vi "rqcBob ServiceNET Read Data.vi"(8 "error in":errorcluster, 11 "rqcBob ServiceNET in":T1) -> (0 "error out":errorcluster, 1 "data valid":bool, 2 "Data":u32[](array[numeric]), 3 "rqcBob ServiceNET out":T1)   [LabVIEW 2018]
uses:
  Custom Controls/rqcBob ServiceNET control.ctl
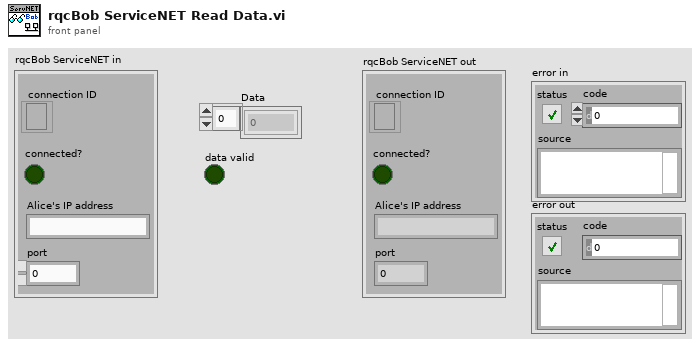
[diagram p1: front panel]
types:
  T1 = typedef "rqcBob ServiceNET control.ctl" = cluster{"connection ID":refnum<k5>, "connected?":bool, "Alice's IP address":string, "port":u16}
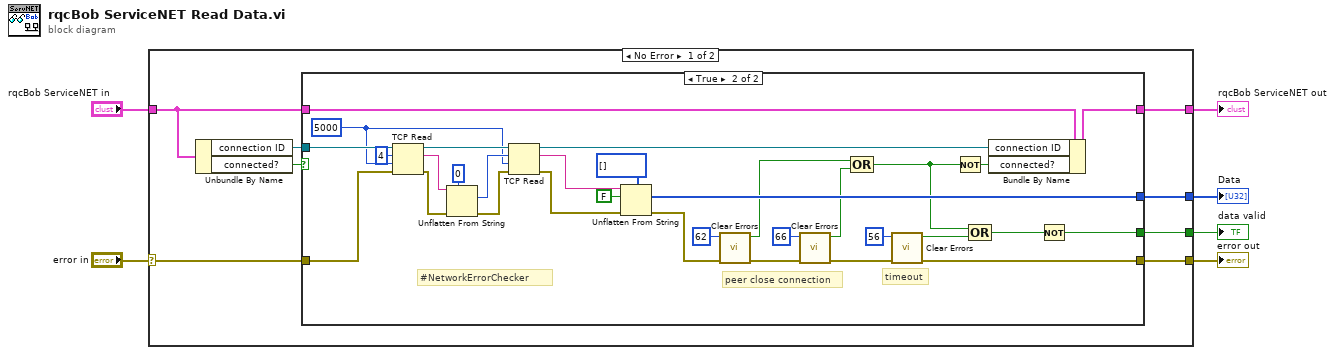
[diagram p0: block diagram]
diagram:
  n1 = case shown="No Error" "error in" {
    selector: "error in" -> [w12 w50]
    tunnel: "rqcBob ServiceNET in" -> [w10 w49]
    tunnel: [w11 w50] -> w4
    tunnel: [w9 w49] -> w3
    tunnel: [w8 _] -> w2
    tunnel: [w7 _] -> w1
    frame No Error {
      n2 = Unbundle By Name(w10) -> ("connection ID"=w13:refnum<k5>, "connected?"=w14:bool)
      n3 = case shown="True" w14 {
        tunnel: w13 -> [_ w46]
        tunnel: w12 -> [w16 w45]
        tunnel: [w16 w24] -> w11
        tunnel: [w15 w47] -> w9
        tunnel: w10 -> [w15 w48]
        tunnel: [_ w32] -> w8
        tunnel: [_ w25] -> w7
        frame False {
        }
        frame True {
          w29 = 5000 ("timeout ms (25000)")
          # "peer close connection"
          # "timeout"
          # "#NetworkErrorChecker"
          n4 = TCP Read(connection ID=w46, bytes to read=4, error in (no error)=w45, 9:w29) -> (connection ID out=w40:refnum<k5>, data out=w43:string, error out=w41:errorcluster)  [unwired: 1 in]
          n5 = Unflatten From String(type=0, binary string=w43, error in (no error)=w41) -> (value=w37:i32, error out=w38:errorcluster)  [unwired: 2 in, 1 out]
          n6 = TCP Read(connection ID=w40, bytes to read=w37, error in (no error)=w38, 9:w29) -> (connection ID out=w39:refnum<k5>, data out=w35:string, error out=w36:errorcluster)  [unwired: 1 in]
          n7 = Unflatten From String(type=u32[] [], binary string=w35, data includes array or string size? (T)=FALSE, error in (no error)=w36) -> (value=w32:u32[], error out=w22:errorcluster)  [unwired: 1 in, 1 out]
          n8 = call <vilib>:"Clear Errors.vi"("error in (no error)"=w22, "specific error code to clear (0: all)"=62) -> ("error out"=w21:errorcluster, "specific error cleared?"=w19:bool)  [unwired: 4 in]
          n9 = call <vilib>:"Clear Errors.vi"("error in (no error)"=w21, "specific error code to clear (0: all)"=66) -> ("error out"=w27:errorcluster, "specific error cleared?"=w20:bool)  [unwired: 4 in]
          n10 = Compound Arithmetic op=OR(w19, w20) -> (w17:bool)
          n11 = call <vilib>:"Clear Errors.vi"("error in (no error)"=w27, "specific error code to clear (0: all)"=56) -> ("error out"=w24:errorcluster, "specific error cleared?"=w26:bool)  [unwired: 4 in]
          n12 = Not(x=w17) -> (.not. x?=w28:bool)
          n13 = Compound Arithmetic op=OR(w17, w26) -> (w18:bool)
          n14 = Bundle By Name(cluster=w48, "connection ID"=w39, "connected?"=w28) -> (w47:T1)
          n15 = Not(x=w18) -> (.not. x?=w25:bool)
        }
      }
    }
    frame Error {
    }
  }
  "error out" <- w4
  "rqcBob ServiceNET out" <- w3
  "Data" <- w2
  "data valid" <- w1
